vi "EcuReset.vi"(5 "LogSuspend":bool, 8 "error in":errorcluster, 10 "Subfunciton":T1(ring)=enum."Soft Reset", 11 "UdsHandleIn":T2={"LogPath"=path "", "LogEnabled"=FALSE, "isOpen"=FALSE, "LogContent"="", "Adapter"="CAN0", "MCanHandle"={"MCanAdapter"=refnum}, "TransmittId"=0, "ReceiveId"=0}) -> (0 "error out":errorcluster, 3 "UdsHandleOut":T2={"LogPath"=path "", "LogEnabled"=FALSE, "isOpen"=FALSE, "LogContent"="", "Adapter"="CAN0", "MCanHandle"={"MCanAdapter"=refnum}, "TransmittId"=0, "ReceiveId"=0})   [LabVIEW 2011, in "Konvolucio MUDS150628.lvlib"]
uses:
  <instrlib>/Konvolucio MUDS150628/Konvolucio MUDS150628.lvlib
  <instrlib>/Konvolucio MUDS150628/Types/UdsHandleType.ctl
  <instrlib>/Konvolucio MCAN120803/Types/MCanHandleType.ctl
  C:/Program Files/National Instruments/LabVIEW 2011/instr.lib/Konvolucio MCAN120803/Private/Konvolucio.MCAN120803.dll
  Konvolucio MCAN120803/Private/Konvolucio.MCAN120803.dll
  <instrlib>/Konvolucio MCAN120803/Konvolucio MCAN120803.lvlib
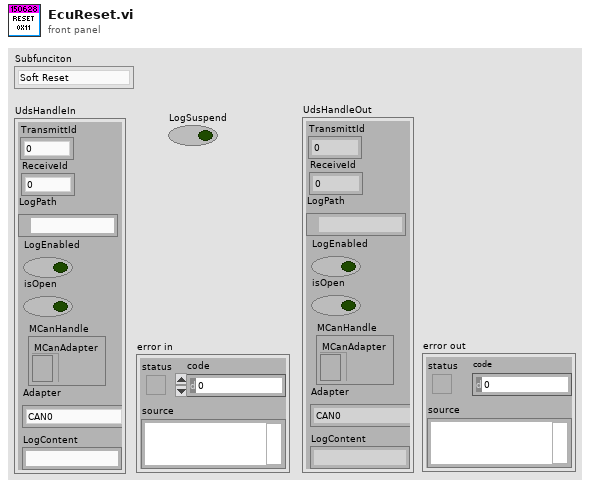
[diagram p1: front panel]
types:
  T1 = enum16{"Hard Reset", "Key Off On Reset", "Soft Reset"}
  T2 = typedef "Konvolucio MUDS150628.lvlib/UdsHandleType.ctl" = cluster{"LogPath":path, "LogEnabled":bool, "isOpen":bool, "LogContent":string, "Adapter":string, "MCanHandle":T3, "TransmittId":u32, "ReceiveId":u32}
  T3 = typedef "Konvolucio MCAN120803.lvlib/MCanHandleType.ctl" = cluster{"MCanAdapter":refnum<k24>}
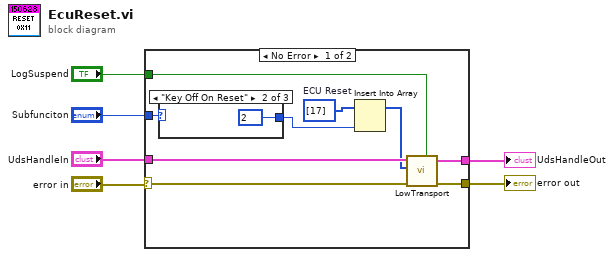
[diagram p0: block diagram]
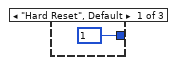
[diagram p2: hidden frame]
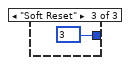
[diagram p3: hidden frame]
diagram:
  n1 = case shown="No Error" "error in" {
    selector: "error in" -> [w14 w20]
    tunnel: "UdsHandleIn" -> [w15 w19]
    tunnel: [w13 w20] -> w4
    tunnel: [w12 w19] -> w3
    tunnel: "LogSuspend" -> [w11 _]
    tunnel: "Subfunciton" -> [w9 _]
    frame No Error {
      w8 = u8[] [17]  # ECU Reset
      n2 = case shown="\"Key Off On Reset\"" w9 {
        tunnel: [1 2 3] -> w7
        frame "Hard Reset", Default {
        }
        frame "Key Off On Reset" {
        }
        frame "Soft Reset" {
        }
      }
      n3 = Insert Into Array(array=w8, new element=w7) -> (w10:u8[])  [unwired: 1 in]
      n4 = call <instrlib>:"LowTransport.vi"("LogSuspend"=w11, "error in"=w14, "Request"=w10, "HandleIn"=w15) -> ("error out"=w13:errorcluster, "HandleOut"=w12:T2)  [unwired: 5 in, 1 out]
    }
    frame Error {
    }
  }
  "error out" <- w4
  "UdsHandleOut" <- w3
